vi "Get Settings Name.vi"(8 "error in (no error)":errorcluster {"code" format="Error %.0f"}, 11 "Printer Settings In":refnum<class "Printer Settings.lvclass">) -> (0 "error out":errorcluster {"code" format="Error %.0f"}, 2 "Name":string, 3 "Printer Settings Out":refnum<class "Printer Settings.lvclass">)   [LabVIEW 2023, in "VIDoc Printer.lvlib" / "Printer Settings.lvclass"]
uses:
  Printer Settings.lvclass
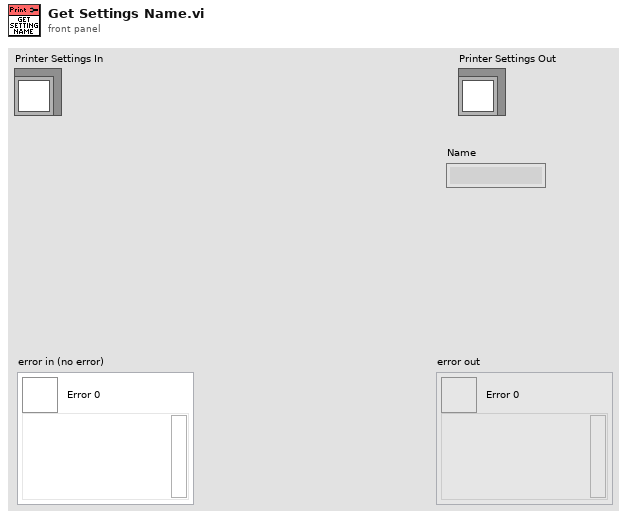
[diagram p1: front panel]
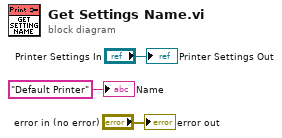
[diagram p0: block diagram]
diagram:
  "error out" <- "error in (no error)"
  "Printer Settings Out" <- "Printer Settings In"
  "Name" <- "Default Printer" ("Name")
